vi "Write_InputRegisters.vi"   [LabVIEW 2016]
uses:
  <vilib>/NI/Current Value Table/Type Defs/File Format.ctl
  <vilib>/NI/Current Value Table/Type Defs/Single Tag.ctl
  <vilib>/NI/Current Value Table/Type Defs/Data Types.ctl
  <vilib>/NI/Current Value Table/Type Defs/Tag Grouping set.ctl
  <vilib>/NI/Current Value Table/DataTypes/U16_Write.vi
  <vilib>/NI/Current Value Table/Type to Enum.vi
  <vilib>/NI/Current Value Table/DataTypes/U16_Type To Enum.vi
  MB_Master_TCP/MB_Master_TCP.lvclass
  C:/Users/PRANAV/Desktop/Modbus_Scada_Main/Modbus_Scada/MB_Master/MB_Master.lvclass
  <vilib>/Utility/file.llb/Read Delimited Spreadsheet (string).vi
  Main_Stop_Global.vi
  <vilib>/NI/Current Value Table/FGVs/CVT Globals.vi
  <vilib>/NI/Current Value Table/FGVs/Tag Memory.vi
  <vilib>/NI/Current Value Table/Memory Block.vi
  <vilib>/NI/Current Value Table/DataTypes/U16_Memory Block.vi
  <vilib>/NI/Current Value Table/Current Value Table.lvlib
  MB Master.lvlib
types:
  T1 = typedef "Current Value Table.lvlib/Tag Grouping set.ctl" = cluster{"Group":string, "Tag Names":string[]}
  T2 = typedef "Current Value Table.lvlib/File Format.ctl" = cluster{"Tags":T3[], "Group Listings":T1[]}
  T3 = typedef "Current Value Table.lvlib/Single Tag.ctl" = cluster{"Data Type":T4, "Name":string, "Value":string, "Description":string}
  T4 = typedef "Current Value Table.lvlib/Data Types.ctl" = enum16{"Double", "Single", "I64", "I32", "I16", "I8", "U64", "U32", "U16", "U8", "String", "Boolean", "Array of U8", "Array of U16", "Array of U32", "Array of U64", "Array of I64", "Array of I32", "Array of I16", "Array of I8", "Array of Double", "Array of Single", "Array of Boolean", "Array of String"}
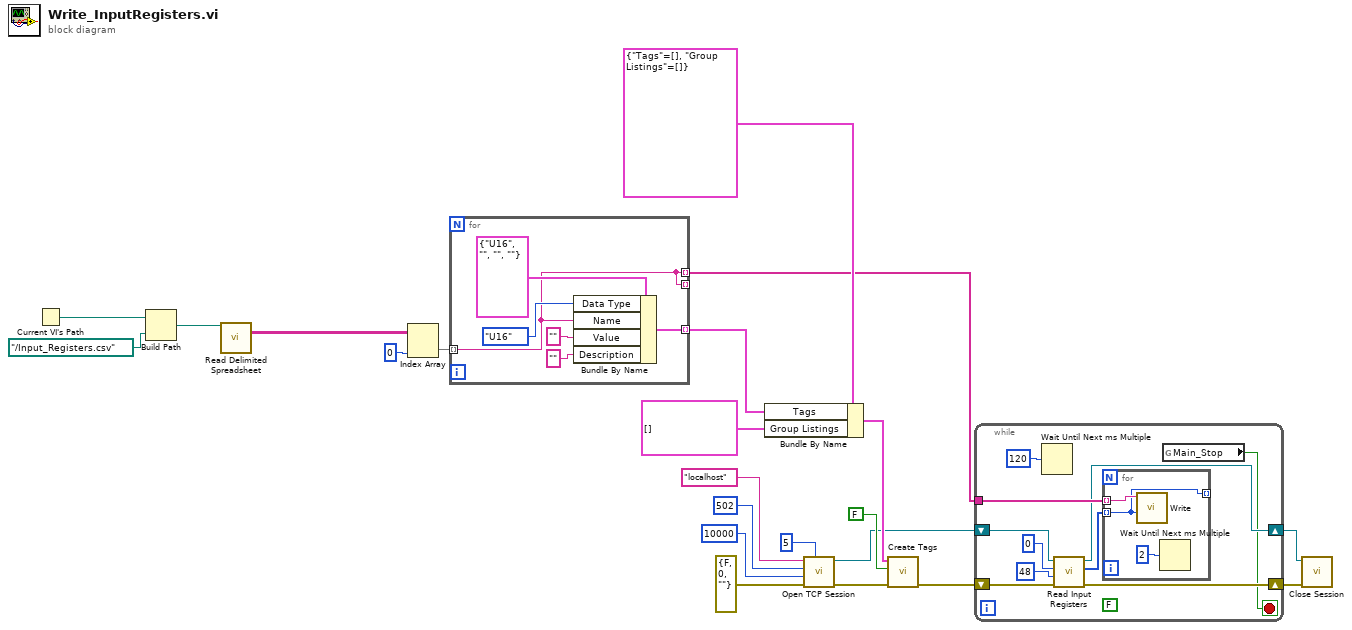
[diagram p0: block diagram]
diagram:
  n1 = Current VI's Path() -> (path=w3:path)
  n2 = Build Path(base path=w3, name or relative path=path "../Input_Registers.csv") -> (appended path=w1:path)
  n3 = call-poly <vilib>:"Read Delimited Spreadsheet.vi"("file path (dialog if empty)"=w1) -> ("all rows"=w12:string[][])  [unwired: 9 in, 5 out]
  n4 = Index Array(array=w12, index (col)=0 ("disabled index (col)")) -> (element=w19:string[])  [unwired: 1 in]
  n5 = for {
    tunnel: w19 -> [w23] mode=indexing
    tunnel: [w28] -> w18 mode=indexing
    tunnel: [w23] -> _ mode=indexing
    tunnel: [w23] -> w5 mode=indexing
    n6 = Bundle By Name(cluster=T3 {"Data Type"=enum."U16", "Name"="", "Value"="", "Description"=""} ("element"), "Data Type"=Data_Types."U16", "Name"=w23, "Value"="", "Description"="") -> (w28:T3)
  }
  n7 = Bundle By Name(cluster=T2 {"Tags"=[], "Group Listings"=[]} ("CVT Tags to Create"), "Tags"=w18, "Group Listings"=T1[] []) -> (w20:T2)
  n8 = call "Open TCP Session.vi"("Slave ID (255)"=u8 5, "error in (no error)"=errorcluster {"status"=FALSE, "code"=0, "source"=""}, "Timeout (10000)"=10000, "Port (502)"=u16 502, "IP Address"="localhost") -> ("error out"=w9:errorcluster, "MB_TCP session"=w6:refnum<class "MB_Master_TCP.lvclass">)  [unwired: 5 in]
  n9 = call <vilib>:"Create Tags.vi"("error in (no error)"=w9, "Clear Table? (F)"=FALSE, "CVT Tags to Create"=w20) -> ("error out"=w8:errorcluster)  [unwired: 8 in]
  n10 = while {
    shift-right: [w33] -> w7
    shift-left: w8 -> [w36]
    shift-right: [w31] -> w4
    shift-left: w6 -> [w37]
    tunnel: w5 -> [w38]
    stop <- w29 stop-if-true
    (unwired) FALSE
    n11 = Wait Until Next ms Multiple(millisecond multiple=u32 120 ("millisecond timer value")) -> ()  [unwired: 1 out]
    n12 = call "Read Input Registers.vi"("error in (no error)"=w36, "quantity"=u16 48, "starting address"=u16 0, "MB session in"=w37) -> ("error out"=w33:errorcluster, "Registers"=w32:u16[], "MB session out"=w31:refnum<class "MB_Master_TCP.lvclass">)  [unwired: 5 in]
    n13 = for {
      tunnel: w38 -> [w41] mode=indexing
      tunnel: [w40] -> _ mode=indexing
      tunnel: w32 -> [w40] mode=indexing
      n14 = call-poly <vilib>:"Write.vi"("Value"=w40, "Tag Name"=w41) -> ()  [unwired: 9 in, 1 out]
      n15 = Wait Until Next ms Multiple(millisecond multiple=u32 2 ("millisecond timer value")) -> ()  [unwired: 1 out]
    }
    n16 = global read "Main_Stop_Global.vi" "Main_Stop"() -> (w29:bool)
  }
  n17 = call-dynamic "Close Session.vi"("error in (no error)"=w7, "MB TCP session"=w4) -> ()  [unwired: 9 in, 1 out]
